vi "MouseZoomSingleY.vi"(6 "YNum":i32=8, 8 "ZoomMode":u16=2, 9 "Coords":T1, 10 "Delta":i32, 11 "XYGraph输入":refnum<vi>) -> ()   [LabVIEW 2015]
uses:
  <vilib>/Utility/miscctls.llb/LVPoint32TypeDef.ctl
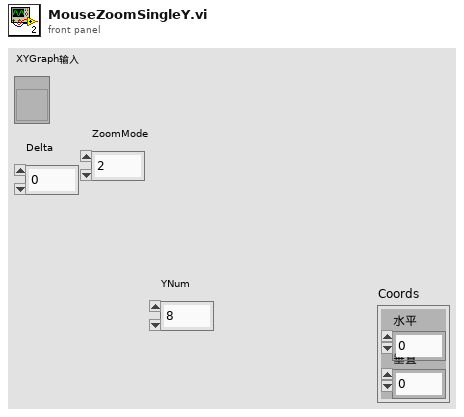
[diagram p1: front panel]
types:
  T1 = typedef "LVPoint32TypeDef.ctl" = cluster{"Horizontal":i32, "Vertical":i32}
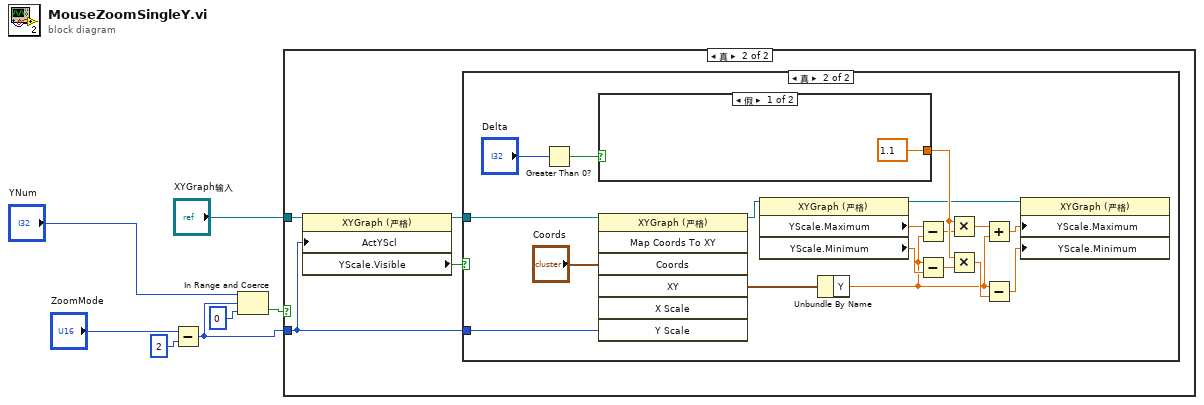
[diagram p0: block diagram]
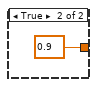
[diagram p4: hidden frame]
diagram:
  n1 = Subtract(x="ZoomMode", y=u16 2) -> (x-y=w4:u16)
  n2 = In Range and Coerce(upper limit="YNum", x=w4, lower limit=0 ("下限")) -> (In Range?=w1:bool)  [unwired: 1 out]
  n3 = case shown="真" w1 {
    tunnel: "XYGraph输入" -> [_ w11]
    tunnel: w4 -> [_ w9]
    frame False {
    }
    frame True {
      n4 = property class="XYGraph (严格)"(reference=w11, "ActYScl"=w9) -> (reference out=w10:refnum<vi>, "YScale.Visible"=w8:bool)  [unwired: 1 in, 1 out]
      n5 = case shown="真" w8 {
        tunnel: w10 -> [_ w13]
        tunnel: w9 -> [_ w12]
        frame False {
        }
        frame True {
          n6 = Greater Than 0?(x="Delta") -> (x > 0?=w29:bool)
          n7 = case shown="假" w29 {
            tunnel: [1.1 0.9] -> w27
            frame False {
            }
            frame True {
            }
          }
          n8 = invoke class="XYGraph (严格)" method="Map Coords To XY"(reference=w13, "Coords"="Coords", "Y Scale"=w12) -> (reference out=w14:refnum<vi>, "XY"=w15:cluster{"X":dbl, "Y":dbl})  [unwired: 4 in, 5 out]
          n9 = property class="XYGraph (严格)"(reference=w14) -> (reference out=w20:refnum<vi>, "YScale.Maximum"=w19:dbl, "YScale.Minimum"=w24:dbl)  [unwired: 1 in, 1 out]
          n10 = Unbundle By Name(w15) -> ("Y"=w17:dbl)
          n11 = Subtract(x=w19, y=w17) -> (x-y=w26:dbl)
          n12 = Subtract(x=w17, y=w24) -> (x-y=w23:dbl)
          n13 = Multiply(x=w27, y=w26) -> (x*y=w25:dbl)
          n14 = Multiply(x=w27, y=w23) -> (x*y=w22:dbl)
          n15 = Add(x=w25, y=w17) -> (x+y=w18:dbl)
          n16 = Subtract(x=w17, y=w22) -> (x-y=w21:dbl)
          n17 = property class="XYGraph (严格)"(reference=w20, "YScale.Maximum"=w18, "YScale.Minimum"=w21) -> ()  [unwired: 1 in, 2 out]
        }
      }
    }
  }
